vi "init_parameters.vi"() -> (3 "Resource name out":string)   [LabVIEW 2018, in "imaginaryStage.lvclass"]
uses:
  imaginaryStage.lvclass
panel:
  in  "OK Button":bool
  in  "Resources name":string
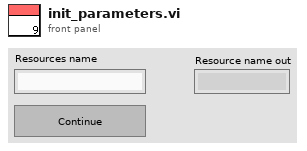
[diagram p1: front panel]
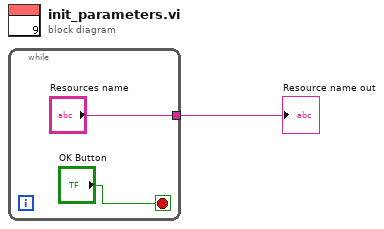
[diagram p0: block diagram]
diagram:
  n1 = while {
    tunnel: ["Resources name"] -> w1
    stop <- "OK Button" stop-if-true
  }
  "Resource name out" <- w1
